vi "DiffDriveTrainSim_GetDynamics.vi"(9 "U":T1, 10 "X":T1, 11 "Info":variant) -> (0 "Error":bool, 3 "XDOT":T1)   [LabVIEW 2019, in "Trajectory_Library.lvlib"]
doc: "Diff Drive Train Sim internal call back function to get dynamics. This is used by the Update function.\n\nInputs:\n - Info -- Extra data variant value containing:\n Matrix A\n Matrix B\n Double CurrentGear\n Double OriginalGear\n Double m_rb \n - X -- X matrix\n - U -- U matrix\n\nOutputs:\n - xDot\n - Error -- If TRUE, an error occured."
uses:
  Trajectory_Library.lvlib
  <vilib>/Analysis/Matrix/Datatypes/RealMatrix.ctl
  <vilib>/Analysis/baseanly.llb/Real A x B.vi
  MatrixHelper_CoerceSize.vi
  <vilib>/Analysis/7linalg.llb/Create Special Matrix.vi
  <vilib>/Analysis/7linalg.llb/Create Special Real Matrix.vi
  <vilib>/Analysis/Matrix/Numeric/Multiply/Multiply - RM,R.vi
  <vilib>/Analysis/Matrix/Numeric/Add/Add - RM,RM.vi
  <vilib>/Analysis/Matrix/NI_Matrix.lvlib
  <vilib>/Analysis/NI_AALBase.lvlib
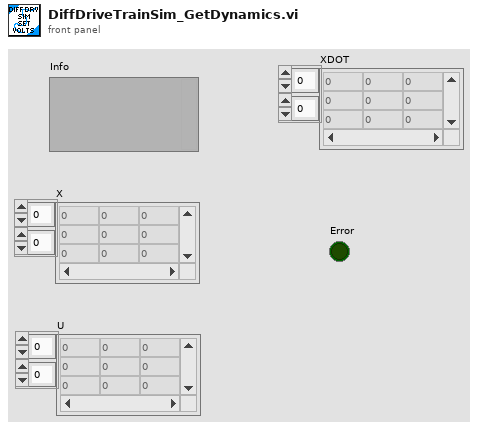
[diagram p1: front panel]
types:
  T1 = typedef "NI_Matrix.lvlib/RealMatrix.ctl" = dbl[][]
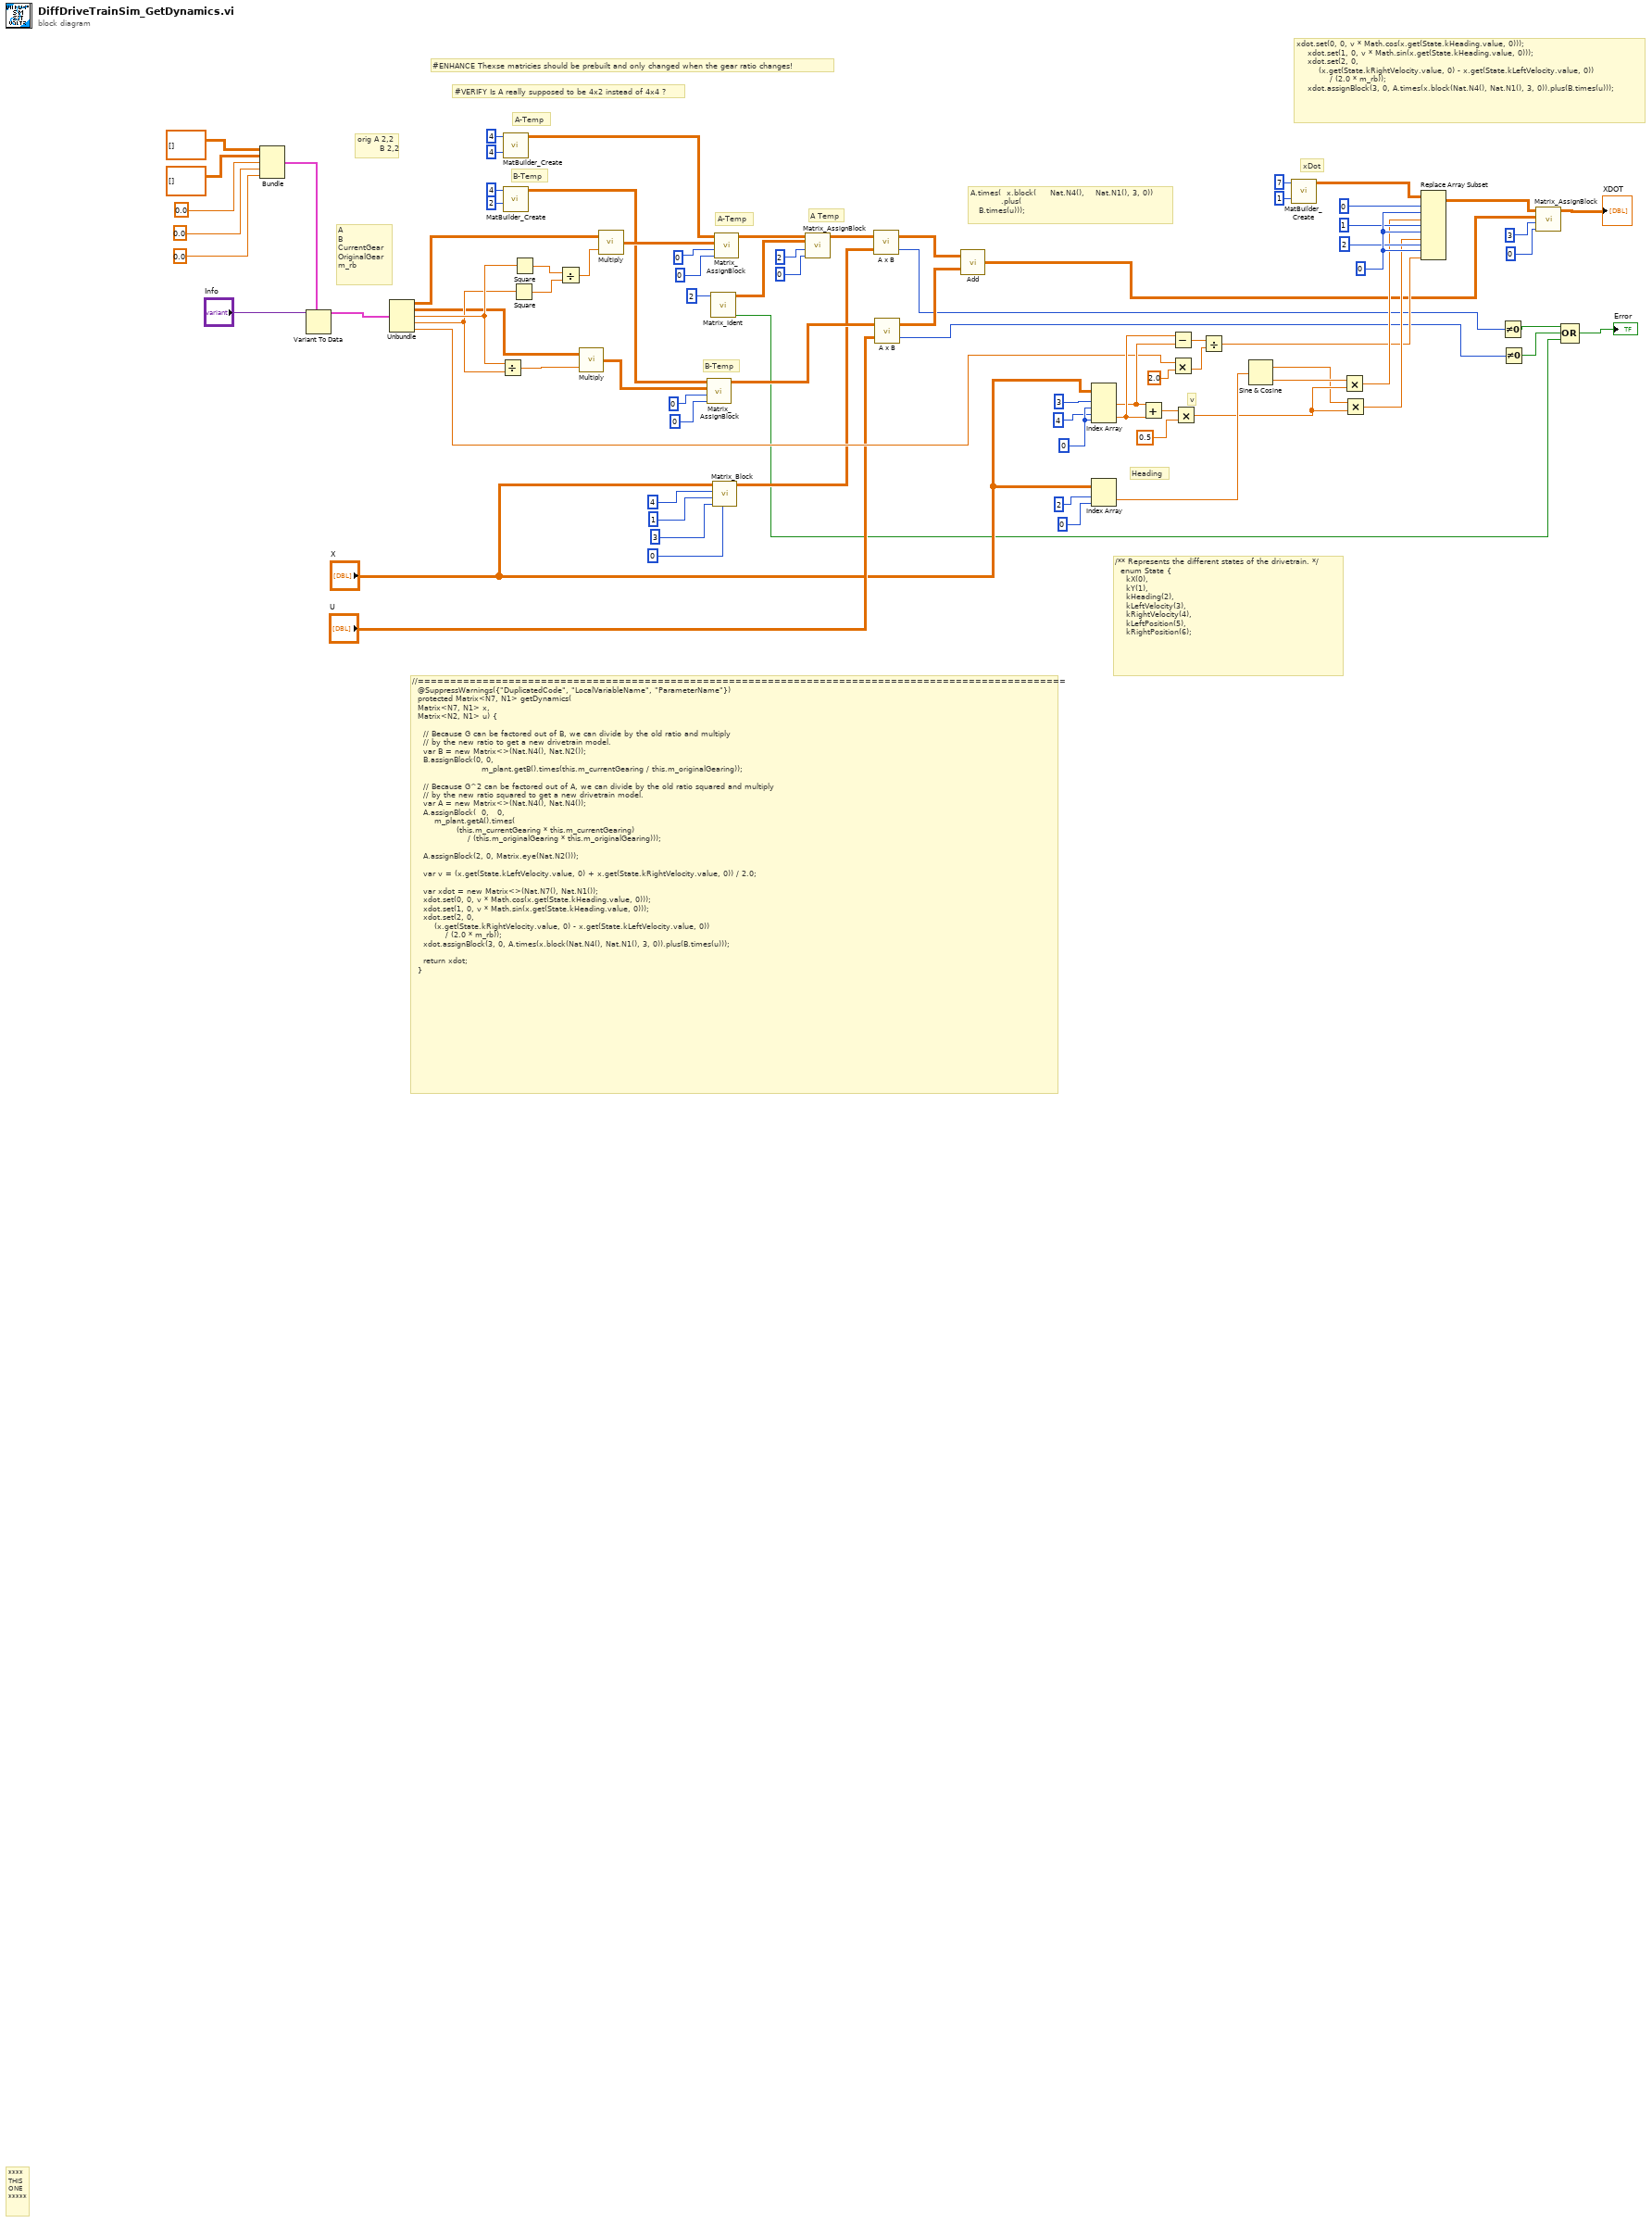
[diagram p0: block diagram]
diagram:
  w53 = 0 ("index (col)")
  w60 = 0 ("index (col)")
  # "B-Temp"
  # "A-Temp"
  # "A.times(  x.block(     Nat.N4(),    Nat.N1(), 3, 0))\n           .plus(  \n   B.times(u)));"
  # "Heading"
  # "v"
  # "xdot.set(0, 0, v * Math.cos(x.get(State.kHeading.value, 0)));\n    xdot.set(1, 0, v * Math.sin(x.get(State.kHeading.value, 0)));\n    xdot.set(2, 0,\n        (x.get(State.kRightVelocity.value, 0) - x.get(State.kLeftVelocity.value, 0))\n            / (2.0 * m_rb));\n    xdot.assignBlock(3, 0, A.times(x.block(Nat.N4(), Nat.N1(), 3, 0)).plus(B.times(u)));"
  # "/** Represents the different states of the drivetrain. */\n  enum State {\n    kX(0),\n    kY(1),\n    kHeading(2),\n    kLeftVelocity(3),\n    kRightVelocity(4),\n    kLeftPosition(5),\n    kRightPosition(6);"
  # "xDot"
  # "#VERIFY Is A really supposed to be 4x2 instead of 4x4 ?"
  # "A Temp"
  # "orig A 2,2\n        B 2,2"
  # "B-Temp"
  # "A-Temp"
  # "A\nB\nCurrentGear\nOriginalGear\nm_rb"
  # "#ENHANCE Thexse matricies should be prebuilt and only changed when the gear ratio changes!"
  # "//====================================================================================================\n  @SuppressWarnings({\"DuplicatedCode\", \"LocalVariableName\", \"ParameterName\"})\n  protected Matrix<N7, N1> getDynamics(\n\t\tMatrix<N7, N1> x, \n\t\tMatrix<N2, N1> u) {\n\n    // Because G can be factored out of B, we can divide by the old ratio and multiply\n    // by the new ratio to get a new drivetrain model.\n    var B = new Matrix<>(Nat.N4(), Nat.N2());\n    B.assignBlock(0, 0, \n\t\t                       m_plant.getB().times(this.m_currentGearing / this.m_originalGearing));\n\n    // Because G^2 can be factored out of A, we can divide by the old ratio squared and multiply\n    // by the new ratio squared to get a new drivetrain model.\n    var A = new Matrix<>(Nat.N4(), Nat.N4());\n    A.assignBlock(  0,   0,\n        m_plant.getA().times(\n                (this.m_currentGearing * this.m_currentGearing)\n                    / (this.m_originalGearing * this.m_originalGearing)));\n\n    A.assignBlock(2, 0, Matrix.eye(Nat.N2()));\n\n    var v = (x.get(State.kLeftVelocity.value, 0) + x.get(State.kRightVelocity.value, 0)) / 2.0;\n\n    var xdot = new Matrix<>(Nat.N7(), Nat.N1());\n    xdot.set(0, 0, v * Math.cos(x.get(State.kHeading.value, 0)));\n    xdot.set(1, 0, v * Math.sin(x.get(State.kHeading.value, 0)));\n    xdot.set(2, 0,\n        (x.get(State.kRightVelocity.value, 0) - x.get(State.kLeftVelocity.value, 0))\n            / (2.0 * m_rb));\n    xdot.assignBlock(3, 0, A.times(x.block(Nat.N4(), Nat.N1(), 3, 0)).plus(B.times(u)));\n\n    return xdot;\n  }"
  # "****\nTHIS\nONE\n*****"
  n1 = Bundle("matrix"=T1 [], "matrix"=T1 [], 0.0, 0.0, 0.0) -> (w69:cluster{"matrix":T1, "matrix":T1, dbl, dbl, dbl})  [unwired: 1 in]
  n2 = Variant To Data(type=w69, Variant="Info") -> (data=w68:cluster{"matrix":T1, "matrix":T1, dbl, dbl, dbl})  [unwired: 1 in, 1 out]
  n3 = Unbundle(w68) -> ("matrix"=w78:T1, "matrix"=w76:T1, w82:dbl, w81:dbl, w39:dbl)
  n4 = Divide(x=w82, y=w81) -> (x/y=w75:dbl)
  n5 = call "MatBuilder_Create.vi"("Columns"=4, "Rows"=4) -> ("output matrix"=w27:T1)  [unwired: 9 in]
  n6 = call "MatBuilder_Create.vi"("Columns"=2, "Rows"=4) -> ("output matrix"=w23:T1)  [unwired: 9 in]
  n7 = Square(x=w81) -> (x^2=w79:dbl)
  n8 = Square(x=w82) -> (x^2=w80:dbl)
  n9 = Divide(x=w80, y=w79) -> (x/y=w77:dbl)
  n10 = call-poly <vilib>:"Multiply.vi"("Real Scalar c"=w75, "Real Matrix A"=w76) -> ("A * c"=w22:T1)
  n11 = call-poly <vilib>:"Multiply.vi"("Real Scalar c"=w77, "Real Matrix A"=w78) -> ("A * c"=w26:T1)
  n12 = call "Matrix_AssignBlock.vi"("StartColumn"=0 ("row N"), "StartRow"=0 ("row 1"), "Other Matrix"=w22, "input matrix"=w23) -> ("output matrix"=w12:T1)  [unwired: 7 in]
  n13 = call "Matrix_Ident.vi"("Size"=2 ("matrix size")) -> ("Error"=w1:bool, "output matrix"=w3:T1)  [unwired: 9 in]
  n14 = call "Matrix_Block.vi"("StartColumn"=0, "StartRow"=3, "Columns"=1, "Rows"=4, "input matrix"="X") -> ("output matrix"=w10:T1)  [unwired: 6 in]
  n15 = call "Matrix_AssignBlock.vi"("StartColumn"=0 ("row N"), "StartRow"=0 ("row 1"), "Other Matrix"=w26, "input matrix"=w27) -> ("output matrix"=w19:T1)  [unwired: 7 in]
  n16 = call "Matrix_AssignBlock.vi"("StartColumn"=0 ("column 1"), "StartRow"=2 ("row 1"), "Other Matrix"=w3, "input matrix"=w19) -> ("output matrix"=w13:T1)  [unwired: 7 in]
  n17 = call-poly <vilib>:"A x B.vi"("B"=w10, "A"=w13) -> ("error"=w33:i32, "A x B"=w34:T1)
  n18 = call-poly <vilib>:"A x B.vi"("B"="U", "A"=w12) -> ("error"=w32:i32, "A x B"=w35:T1)
  n19 = call-poly <vilib>:"Add.vi"("Real Matrix B"=w35, "Real Matrix A"=w34) -> ("A + B"=w5:T1)
  n20 = Index Array(array="X", index (row) #1=3 ("index (row)"), index (col) #1=w60, index (row) #2=4 ("index (row)"), index (col) #2=w60) -> (element #1=w43:dbl, element #2=w44:dbl)
  n21 = Index Array(array="X", index (row)=2, index (col)=0) -> (element=w49:dbl)
  n22 = Add(x=w43, y=w44) -> (x+y=w58:dbl)
  n23 = Subtract(x=w44, y=w43) -> (x-y=w38:dbl)
  n24 = Multiply(x=w39, y=2.0) -> (x*y=w41:dbl)
  n25 = Multiply(x=w58, y=0.5) -> (x*y=w48:dbl)
  n26 = Divide(x=w38, y=w41) -> (x/y=w37:dbl)
  n27 = Sine & Cosine(0:w49) -> (1:w28:dbl, 2:w47:dbl)
  n28 = call "MatBuilder_Create.vi"("Columns"=1, "Rows"=7) -> ("output matrix"=w54:T1)  [unwired: 9 in]
  n29 = Multiply(x=w47, y=w48) -> (x*y=w46:dbl)
  n30 = Multiply(x=w28, y=w48) -> (x*y=w45:dbl)
  n31 = Replace Array Subset(array=w54, new element #1=w46, index (row) #1=0 ("disabled index (row)"), index (col) #1=w53, new element #2=w45, index (row) #2=1 ("disabled index (row)"), index (col) #2=w53, new element #3=w37, index (row) #3=2 ("disabled index (row)"), index (col) #3=w53) -> (w16:T1)
  n32 = Not Equal To 0?(x=w33) -> (x != 0?=w31:bool)
  n33 = Not Equal To 0?(x=w32) -> (x != 0?=w30:bool)
  n34 = call "Matrix_AssignBlock.vi"("StartColumn"=0 ("row N"), "StartRow"=3 ("row N"), "Other Matrix"=w5, "input matrix"=w16) -> ("output matrix"=→"XDOT":T1)  [unwired: 7 in]
  n35 = Compound Arithmetic op=OR(w31, w30, w1) -> (→"Error":bool)
